vi "Has Error.vi"(8 "error in (no error)":errorcluster, 11 "MDS Command in":T1) -> (0 "error out":errorcluster, 3 "MDS Command out":T1)   [LabVIEW 2019, in "Controller.lvlib"]
uses:
  Controller.lvlib
  MDS Command.ctl
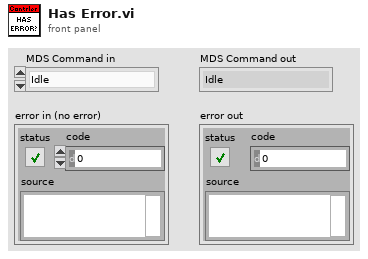
[diagram p1: front panel]
types:
  T1 = typedef "Controller.lvlib/MDS Command.ctl" = enum16{"Idle", "Open", "Set VMode", "Set IMode", "Get Frequency", "Set Frequency", "Get Power", "Set Power (dBm)", "Set Power (%)", "Get Switch", "Switch Channel", "Store", "Wait for Prompt", "Wait for State", "Reset", "Error", "Close", "Stop"}
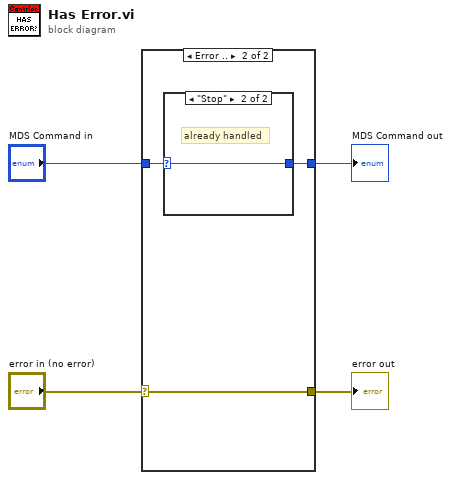
[diagram p0: block diagram]
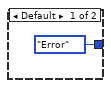
[diagram p3: hidden frame]
diagram:
  n1 = case shown="Error .." "error in (no error)" {
    selector: "error in (no error)" -> [w6 w9]
    tunnel: [w6 w9] -> w3
    tunnel: [w5 w7] -> w2
    tunnel: "MDS Command in" -> [w5 w8]
    frame No Error {
    }
    frame Error {
      n2 = case shown="\"Stop\"" w8 {
        selector: w8 -> [_ w11]
        tunnel: [MDS_Command."Error" ("MDS Command in") w11] -> w7
        frame Default {
        }
        frame "Stop" {
          # "already handled"
        }
      }
    }
  }
  "error out" <- w3
  "MDS Command out" <- w2
